vi "SanitiseADAMChStrings.vi"(11 "Ch Discription in":T1 {"Duty" format="%.0b"; "D" format="%#_5g"; "C" format="%#_5g"; "B" format="%#_5g"; "A" format="%#_5g"}) -> (3 "Ch Discription out":T1 {"Duty" format="%.0b"; "D" format="%#_5g"; "C" format="%#_5g"; "B" format="%#_5g"; "A" format="%#_5g"})   [LabVIEW 2015]
doc: "Remove Returns (\\r) Linefeeds (\\n) and Tabs (\\t) from Name, Comments and String fileds of ADAM channel description cluster."
uses:
  ADAM Client/Sub VIs/ADAM Controls/Ch_description_ADAM.ctl
  ADAM Client/Sub VIs/ADAM Controls/Module_type_ADAM.ctl
  ADAM Client/Sub VIs/ADAM Controls/Function_ADAM.ctl
  ADAM Client/Sub VIs/ADAM Controls/Channel_State.ctl
  ADAM Client/Sub VIs/ADAM Controls/Calib_type_ADAM.ctl
  ADAM Client/Sub VIs/ADAM Controls/Address.ctl
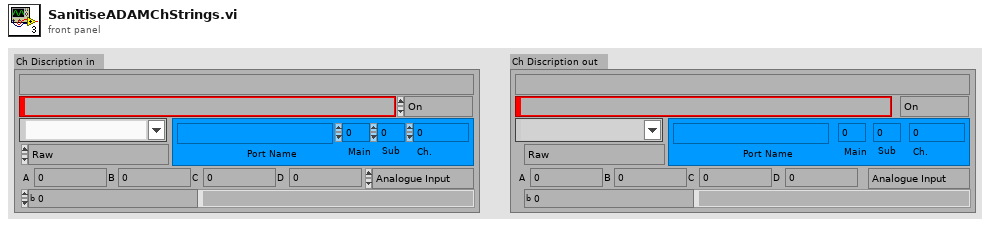
[diagram p1: front panel]
types:
  T1 = typedef "Ch_description_ADAM.ctl" = cluster{"Ch Name":string, "Type":T2, "Function":T3, "Ch State":T4, "Calibration type":T5, "A":dbl, "B":dbl, "C":dbl, "D":dbl, "Comments":string, "Address":T6, "String":string, "Duty":u16}
  T2 = typedef "Module_type_ADAM.ctl" = string
  T3 = typedef "Function_ADAM.ctl" = enum16{"Analogue Input", "Digital Input", "Event counter", "Event rate", "Analogue Output", "Digital Output", "Relay Output"}
  T4 = typedef "Channel_State.ctl" = enum16{"On", "Off", "Always On", "Always Off"}
  T5 = typedef "Calib_type_ADAM.ctl" = enum16{"Raw", "Bx + A", "Cx^2 + Bx + A", "Dx^3 + Cx^2 + Bx + A", "In Band", "Hi-Tec Q", "Hi-Tec M_dot", "Text"}
  T6 = typedef "Address.ctl" = cluster{"Main":i32, "Ch.":i32, "Sub":i32, "Port Name":string}
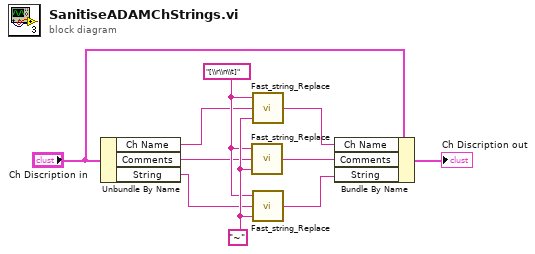
[diagram p0: block diagram]
diagram:
  w5 = "~" ("Replace match with:")
  w4 = "[\\r\\n\\t]" ("regular expression")
  n1 = Unbundle By Name("Ch Discription in") -> ("Ch Name"=w1:string, "Comments"=w2:string, "String"=w3:string)
  n2 = call "Fast_string_Replace.vi"("Replace match with:"=w5, "Input String"=w2, "regular expression"=w4) -> ("Output String"=w8:string)  [unwired: 1 in, 1 out]
  n3 = call "Fast_string_Replace.vi"("Replace match with:"=w5, "Input String"=w1, "regular expression"=w4) -> ("Output String"=w7:string)  [unwired: 1 in, 1 out]
  n4 = call "Fast_string_Replace.vi"("Replace match with:"=w5, "Input String"=w3, "regular expression"=w4) -> ("Output String"=w9:string)  [unwired: 1 in, 1 out]
  n5 = Bundle By Name(cluster="Ch Discription in", "Ch Name"=w7, "Comments"=w8, "String"=w9) -> (→"Ch Discription out":T1)
